vi "RSZVB Revision Query.vi"(8 "error in (no error)":errorcluster {"code" format="%.0x"}, 11 "VISA session":refnum<visa-resource-name>) -> (0 "error out":errorcluster {"code" format="%.0x"}, 1 "Instrument Firmware Revision":string, 2 "Instrument Driver Revision":string, 3 "dup VISA session":refnum<visa-resource-name>)   [LabVIEW 2011]
doc: "This VI queries the current instrument firmware revision and instrument driver revision."
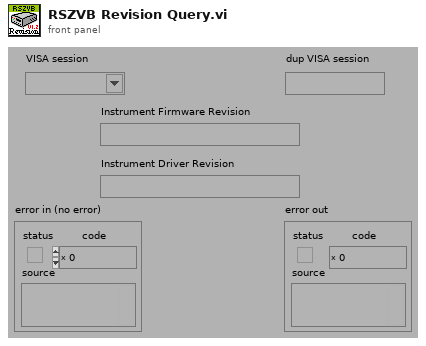
[diagram p1: front panel]
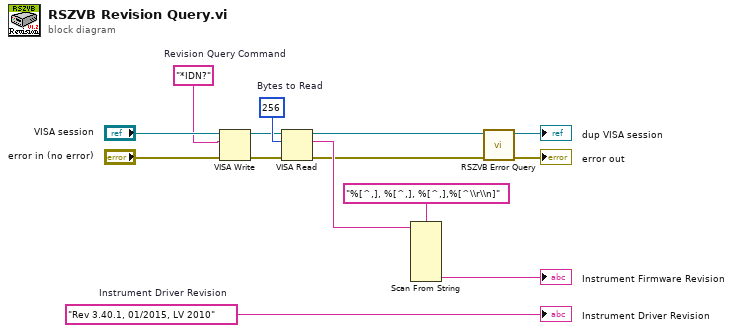
[diagram p0: block diagram]
diagram:
  w7 = "*IDN?"  # Revision Query Command
  w10 = u32 256  # Bytes to Read
  w14 = "Rev 3.40.1, 01/2015, LV 2010"  # Instrument Driver Revision
  n1 = VISA Write(VISA resource name="VISA session", write buffer=w7, error in (no error)="error in (no error)") -> (VISA resource name out=w9:refnum<visa-resource-name>, error out=w8:errorcluster)  [unwired: 1 out]
  n2 = VISA Read(VISA resource name=w9, byte count=w10, error in (no error)=w8) -> (VISA resource name out=w3:refnum<visa-resource-name>, read buffer=w6:string, error out=w4:errorcluster)  [unwired: 1 out]
  n3 = Scan From String(format string="%[^,], %[^,], %[^,],%[^\\r\\n]", input string=w6) -> (output 4=→"Instrument Firmware Revision":string)  [unwired: 9 in, 3 out]
  n4 = call "RSZVB Error Query.vi"("error in (no error)"=w4, "VISA session"=w3) -> ("error out"=→"error out":errorcluster, "dup VISA session"=→"dup VISA session":refnum<visa-resource-name>)  [unwired: 6 in, 2 out]
  "Instrument Driver Revision" <- w14
